vi "Generate Trace for Stopped Time-Delayed Message.vi"(10 "Delivery Notifier":refnum<notifier>) -> ()   [LabVIEW 2020, in "Actor Framework.lvlib"]
doc: "Generates a DETT User Generated Trace for a time-delayed message transmitting its final iteration."
uses:
  Actor Framework.lvlib
  Time-Delayed Send Message/Time-Delay Override Options.ctl
  Support/TDM Registration Mode.ctl
  Support/Localized Strings.vi
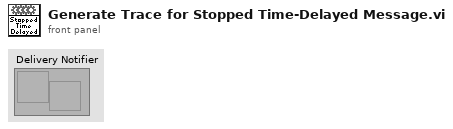
[diagram p1: front panel]
types:
  T1 = typedef "Actor Framework.lvlib/TDM Registration Mode.ctl" = enum16{"Register TDM", "Get ID", "Get Notifier", "Deregister TDM"}
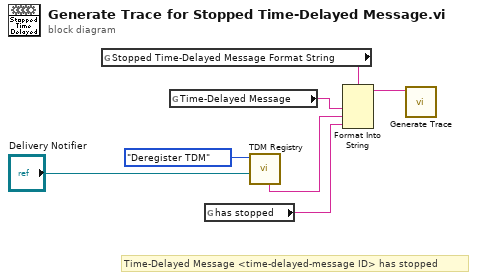
[diagram p0: block diagram]
diagram:
  # "Time-Delayed Message <time-delayed-message ID> has stopped"
  n1 = global read "Localized Strings.vi" "Stopped Time-Delayed Message Format String"() -> (w2:string)
  n2 = global read "Localized Strings.vi" "Time-Delayed Message"() -> (w7:string)
  n3 = global read "Localized Strings.vi" "has stopped"() -> (w6:string)
  n4 = call "TDM Registry.vi"("Delivery Notifier"="Delivery Notifier", "Action"=TDM_Registration_Mode."Deregister TDM") -> ("TDM Alias Out"=w3:string)  [unwired: 5 in, 4 out]
  n5 = Format Into String(format string=w2, w7, w3, w6) -> (resulting string=w1:string)  [unwired: 2 in, 1 out]
  n6 = call "Generate Trace.vi"("String"=w1) -> ()  [unwired: 11 in]
